vi "PH_Beamline_Common.set Waveplate.vi"(1 "Visible (true)":bool=TRUE, 2 "CtlRef":refnum<vi>, 3 "Alignment (vertical)":T1=enum."vertical", 4 "GUI Instance does not exist or here?":bool, 5 "error in (no error)":errorcluster) -> (19 "error out":errorcluster)   [LabVIEW 2014, in "PH_Beamline_Common.lvlib"]
uses:
  PH_Beamline_Common.lvlib
  PH_Common/Picture/PH_Picture.Alignment.ctl
  PH_Common/PH_Common.lvlib
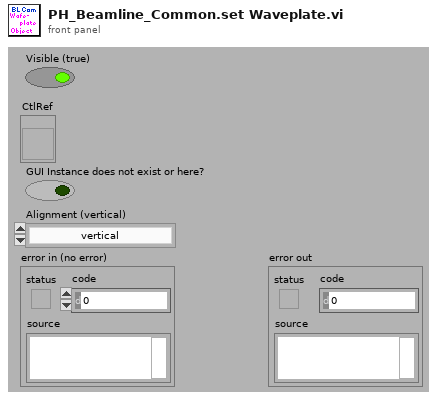
[diagram p1: front panel]
types:
  T1 = typedef "PH_Common.lvlib/PH_Picture.Alignment.ctl" = enum16{"neutral", "left", "right", "up", "down", "vertical", "horizontal", "left down to right up", "left up to right down"}
  T2 = cluster{"left":i16, "top":i16, "right":i16, "bottom":i16}
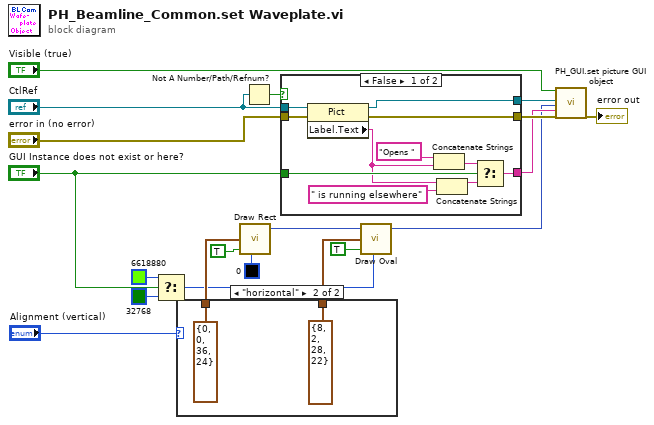
[diagram p0: block diagram]
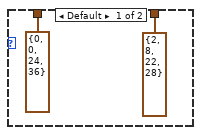
[diagram p2: hidden frame]
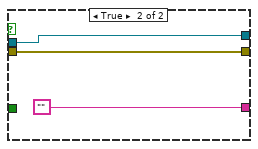
[diagram p3: hidden frame]
diagram:
  n1 = Select(t=u32 6618880, s="GUI Instance does not exist or here?", f=u32 32768 ("Color Box")) -> (s? t:f=w7:u32)
  n2 = case shown="\"horizontal\"" "Alignment (vertical)" {
    tunnel: [T2 {"left"=0, "top"=0, "right"=24, "bottom"=36} ("rect") T2 {"left"=0, "top"=0, "right"=36, "bottom"=24} ("rect")] -> w12
    tunnel: [T2 {"left"=2, "top"=8, "right"=22, "bottom"=28} ("rect") T2 {"left"=8, "top"=2, "right"=28, "bottom"=22} ("rect")] -> w5
    frame Default {
    }
    frame "horizontal" {
    }
  }
  n3 = call <vilib>:"Draw Rect.vi"("rect"=w12, "fill?(F)"=TRUE, "color(black)"=u32 0) -> ("new picture"=w8:picture)  [unwired: 6 in]
  n4 = Not A Number/Path/Refnum?(number/path/refnum="CtlRef") -> (NaN/Path/Refnum?=w14:bool)
  n5 = case shown="False" w14 {
    tunnel: "CtlRef" -> [w34 w38]
    tunnel: "error in (no error)" -> [w33 w37]
    tunnel: [w32 w38] -> w17
    tunnel: [w31 w37] -> w16
    tunnel: [w28 ""] -> w15
    tunnel: "GUI Instance does not exist or here?" -> [w30 _]
    frame False {
      n6 = property class="Pict"(reference=w34, error in=w33) -> (reference out=w32:refnum<vi>, error out=w31:errorcluster, "Label.Text"=w27:string)
      n7 = Concatenate Strings("Opens " ("string"), w27) -> (w29:string)
      n8 = Concatenate Strings(w27, " is running elsewhere" ("string")) -> (w25:string)
      n9 = Select(t=w29, s=w30, f=w25) -> (s? t:f=w28:string)
    }
    frame True {
    }
  }
  n10 = call <vilib>:"Draw Oval.vi"("picture"=w8, "rect"=w5, "fill?(F)"=TRUE, "color(black)"=w7) -> ("new picture"=w6:picture)  [unwired: 5 in]
  n11 = call "PH_GUI.set picture GUI object.vi"("Visible (true)"="Visible (true)", "CtlRef"=w17, "Picture"=w6, "Tip Strip (\"\")"=w15, "error in (no error)"=w16) -> ("error out"=→"error out":errorcluster)  [unwired: 14 in]
